vi "PictToArray28x28.vi"(3 "error in (no error)":errorcluster, 4 "Draw Area Size":cluster{"Width":u32, "Height":u32}, 5 "Picture":picture) -> (0 "error out":errorcluster, 1 "image array":u8[](array[numeric]) format="%.0x", 2 "Array":dbl[][](array[numeric]))   [LabVIEW 2022 SP3]
uses:
  <vilib>/Analysis/baseanly.llb/Mean (DBL).vi
  <vilib>/Analysis/NI_AALBase.lvlib
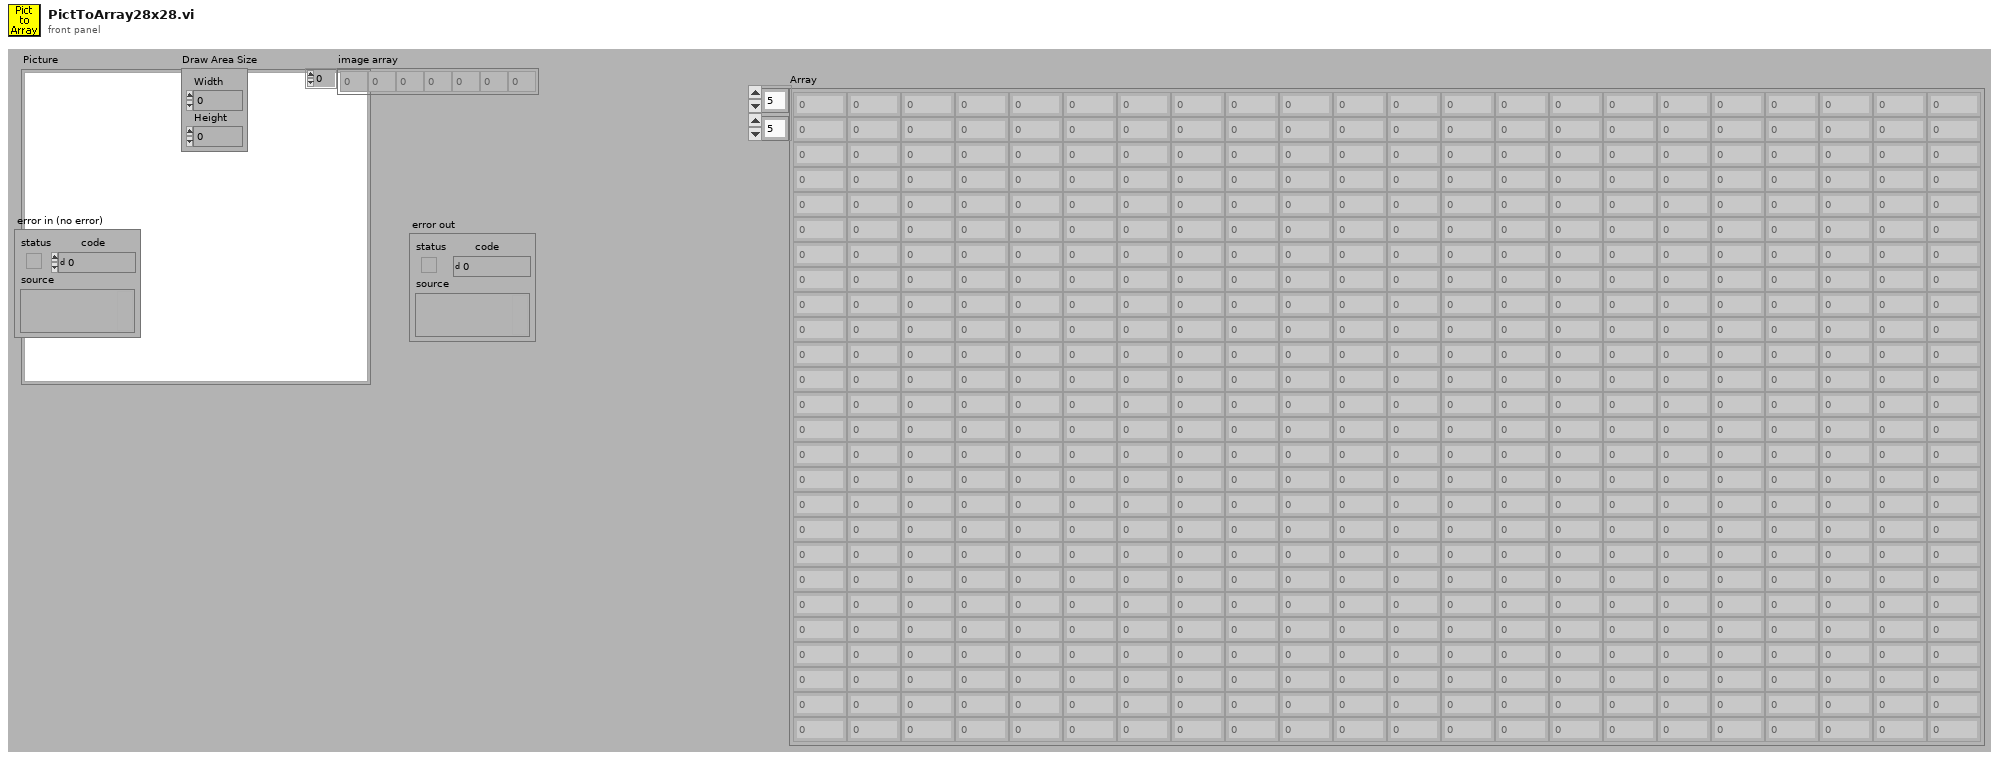
[diagram p1: front panel]
types:
  T1 = typedef "LVBoundsTypeDef.ctl" = cluster{"Width":u32, "Height":u32}
  T2 = typedef "imagedata.ctl" = cluster{"image type":i32, "image depth":i32, "image":u8[], "mask":u8[], "colors":u32[], "Rectangle":cluster{"left":i16, "top":i16, "right":i16, "bottom":i16}}
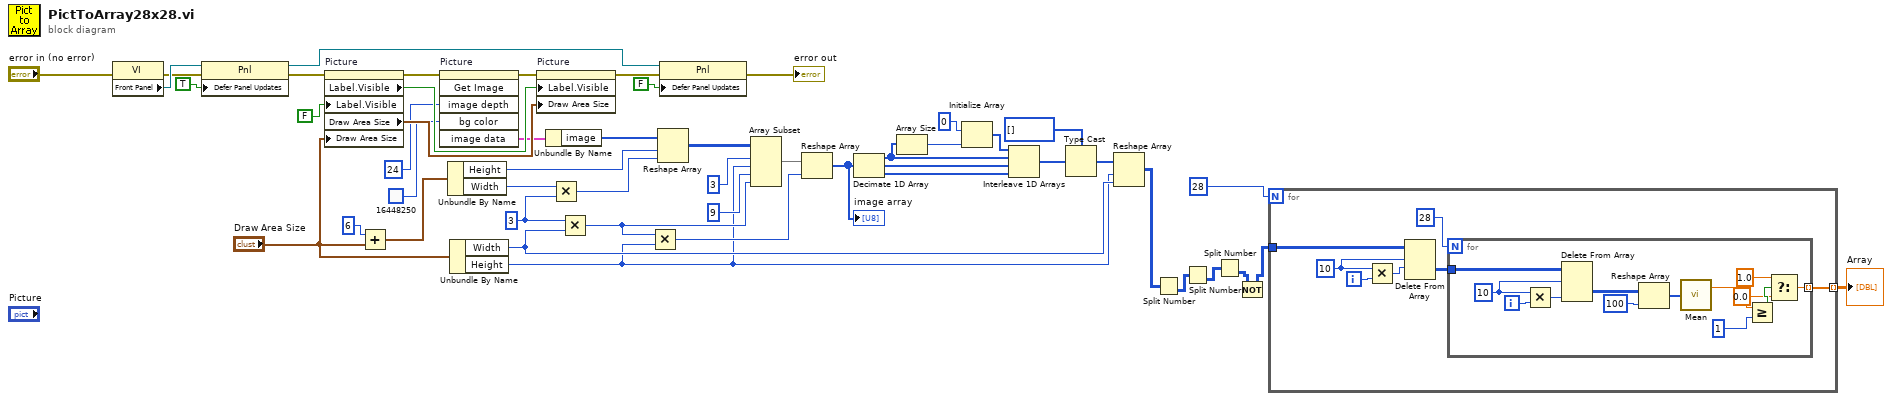
[diagram p0: block diagram]
diagram:
  w29 = u32 3 ("Width")
  n1 = property on="Property Node" class="VI"(error in="error in (no error)") -> (error out=w43:errorcluster, "Front Panel"=w47:refnum<vi>)  [unwired: 1 in, 1 out]
  n2 = property class="Pnl"(reference=w47, error in=w43, "Defer Panel Updates"=TRUE) -> (reference out=w41:refnum<vi>, error out=w42:errorcluster)
  n3 = property on="Picture" class="Pict"(error in=w42, "Label.Visible"=FALSE, "Draw Area Size"="Draw Area Size") -> (error out=w11:errorcluster, "Label.Visible"=w49:bool, "Draw Area Size"=w48:T1)  [unwired: 1 in, 1 out]
  n4 = Add(x=u32 6 ("Width"), y="Draw Area Size") -> (x+y=w36:cluster{"Width":u32, "Height":u32})
  n5 = invoke on="Picture" class="Pict" method="Get Image"(error in=w11, "image depth"=24, "bg color"=u32 16448250 ("Background Color")) -> (error out=w10:errorcluster, "image data"=w13:T2)  [unwired: 3 in, 4 out]
  n6 = Unbundle By Name(w36) -> ("Height"=w31:u32, "Width"=w30:u32)
  n7 = Unbundle By Name("Draw Area Size") -> ("Width"=w18:u32, "Height"=w17:u32)
  n8 = property on="Picture" class="Pict"(error in=w10, "Label.Visible"=w49, "Draw Area Size"=w48) -> (error out=w44:errorcluster)  [unwired: 1 in, 1 out]
  n9 = Unbundle By Name(w13) -> ("image"=w9:u8[])
  n10 = Multiply(x=w30, y=w29) -> (x*y=w35:u32)
  n11 = Multiply(x=w29, y=w18) -> (x*y=w32:u32)
  n12 = Multiply(x=w32, y=w17) -> (x*y=w38:u32)
  n13 = Reshape Array(w9, w31, w35) -> (w39:u8[][])
  n14 = property class="Pnl"(reference=w41, error in=w44, "Defer Panel Updates"=FALSE) -> (error out=→"error out":errorcluster)  [unwired: 1 out]
  n15 = Array Subset(array=w39, index (row)=3 ("index"), length (row)=w17, index (col)=9 ("index"), length (col)=w32) -> (w23:u8[][])
  n16 = Reshape Array(w23, w38) -> (w26:u8[])
  "image array" <- w26
  n17 = Decimate 1D Array(w26) -> (w22:u8[], w24:u8[], w25:u8[])
  n18 = Array Size(array=w22) -> (size(s)=w20:i32)
  n19 = Initialize Array(u8 0, w20) -> (w19:u8[])
  n20 = Interleave 1D Arrays(w19, w22, w24, w25) -> (w16:u8[])
  n21 = Type Cast(type=u32[] [], x=w16) -> (*(type *) &x=w14:u32[])
  n22 = Reshape Array(w14, w17, w18) -> (w5:u32[][])
  n23 = Split Number(x=w5) -> (lo(x)=w4:u16[][])  [unwired: 1 out]
  n24 = Split Number(x=w4) -> (lo(x)=w3:u8[][])  [unwired: 1 out]
  n25 = Split Number(x=w3) -> (lo(x)=w2:u8[][])  [unwired: 1 out]
  n26 = Not(x=w2) -> (.not. x?=w1:u8[][])
  n27 = for {
    N: 28 -> [_]
    tunnel: w1 -> [w57]
    tunnel: [w51] -> w6 mode=indexing
    i -> [w56]
    w55 = 10 ("length")
    n28 = Multiply(x=w55, y=w56) -> (x*y=w54:i32)
    n29 = Delete From Array(array=w57, length=w55, index (row)=w54) -> (deleted portion=w53:u8[][])  [unwired: 1 in, 1 out]
    n30 = for {
      N: 28 -> [_]
      tunnel: w53 -> [w68]
      tunnel: [w61] -> w51 mode=indexing
      i -> [w69]
      w70 = 10 ("length")
      n31 = Multiply(x=w70, y=w69) -> (x*y=w67:i32)
      n32 = Delete From Array(array=w68, length=w70, index (col)=w67) -> (deleted portion=w66:u8[][])  [unwired: 1 in, 1 out]
      n33 = Reshape Array(w66, 100 ("dimension size")) -> (w64:u8[])
      n34 = call-poly <vilib>:"Mean.vi"("X"=w64) -> ("mean"=w62:dbl)  [unwired: 1 out]
      n35 = Greater Or Equal?(x=w62, y=u8 1) -> (x >= y?=w60:bool)
      n36 = Select(t=1.0, s=w60, f=0.0) -> (s? t:f=w61:dbl)
    }
  }
  "Array" <- w6
